vi "Controller Apply Soft Configuration.vi"(8 "error in (no error)":errorcluster, 11 "FOFB Configuration":T1={"FOFB Parameters"={"Network"={"FOFB Controller IP"="", "LNLS Control Network IP"="", "LNLS Control Network Power Supplies TCP Port"=0, "LNLS Control Network FOFB Configuration TCP Port"=0, "LNLS Control Network BPMs TCP Port"=0, "Monitoring Data TCP Port"=0, "Fast Archiver TCP Port"=0, "Fast Command TCP Port"=0, "TCP Listening Timeout"=0}, "Fast Acquisition"={"Sampling Period"=0, "Data Buffer Size"=0, "Monitoring Period"=0}, "Acquisition Network"=[], "Actuation Network"=[]}, "Number of Acquisition Chassis"=0, "Number of Actuation Chassis"=0, "Number of BPM Readings"=0, "BPM Reading Names"=[], "Selected BPM Readings"=[0, 1, 2, 3, 4, 5, 6, 7, 8, 9, 10, 11, 12, 13, 14, 15, 16, 17, 18, 19, 20, 21, 22, 23, 24, 25, 26, 27, 28, 29, 30, 31, 32, 33, 34, 35, 36, 37, 38, 39, 40, 41, 42, 43, 44, 45, 46, 47, 48, 49], "Number of Correctors"=0, "Corrector Names"=[], "Selected Correctors"=[0, 1, 2, 3, 4, 5, 6, 7, 8, 9, 10, 11, 12, 13, 14, 15, 16, 17, 18, 19, 20, 21, 22, 23, 24, 25, 26, 27, 28, 29, 30, 31, 32, 33, 34, 35, 36, 37, 38, 39, 40, 41, 42, 43, 44, 45, 46, 47, 48, 49], "Response Matrix"=[], "Reference Orbit"=[], "Correction Matrix"=[], "FPGA Filter Sets"=[], "Acquisition Chassis Names"=[], "Actuation Chassis Names"=[], "Acquisition Variables"=[], "Actuation Variables"=[], "PS Matrix Mapping"=[], "Inverse PS Matrix Mapping"=[], "BPM Matrix Mapping"=[], "Inverse BPM Matrix Mapping"=[], "BPM Planes"=[], "Corrector Planes"=[]}) -> (0 "error out":errorcluster, 3 "FOFB Configuration":T1={"FOFB Parameters"={"Network"={"FOFB Controller IP"="", "LNLS Control Network IP"="", "LNLS Control Network Power Supplies TCP Port"=0, "LNLS Control Network FOFB Configuration TCP Port"=0, "LNLS Control Network BPMs TCP Port"=0, "Monitoring Data TCP Port"=0, "Fast Archiver TCP Port"=0, "Fast Command TCP Port"=0, "TCP Listening Timeout"=0}, "Fast Acquisition"={"Sampling Period"=0, "Data Buffer Size"=0, "Monitoring Period"=0}, "Acquisition Network"=[], "Actuation Network"=[]}, "Number of Acquisition Chassis"=0, "Number of Actuation Chassis"=0, "Number of BPM Readings"=0, "BPM Reading Names"=[], "Selected BPM Readings"=[0, 1, 2, 3, 4, 5, 6, 7, 8, 9, 10, 11, 12, 13, 14, 15, 16, 17, 18, 19, 20, 21, 22, 23, 24, 25, 26, 27, 28, 29, 30, 31, 32, 33, 34, 35, 36, 37, 38, 39, 40, 41, 42, 43, 44, 45, 46, 47, 48, 49], "Number of Correctors"=0, "Corrector Names"=[], "Selected Correctors"=[0, 1, 2, 3, 4, 5, 6, 7, 8, 9, 10, 11, 12, 13, 14, 15, 16, 17, 18, 19, 20, 21, 22, 23, 24, 25, 26, 27, 28, 29, 30, 31, 32, 33, 34, 35, 36, 37, 38, 39, 40, 41, 42, 43, 44, 45, 46, 47, 48, 49], "Response Matrix"=[], "Reference Orbit"=[], "Correction Matrix"=[], "FPGA Filter Sets"=[], "Acquisition Chassis Names"=[], "Actuation Chassis Names"=[], "Acquisition Variables"=[], "Actuation Variables"=[], "PS Matrix Mapping"=[], "Inverse PS Matrix Mapping"=[], "BPM Matrix Mapping"=[], "Inverse BPM Matrix Mapping"=[], "BPM Planes"=[], "Corrector Planes"=[]})   [LabVIEW 2011, in "Controller VIs.lvlib"]
doc: "Performs tasks related with the FOFB configuration which does not require interrupting controller execution (ex.: load response matrix and reference orbit from file, calculate correction matrix, etc)."
uses:
  Controller VIs.lvlib
  Types Definitions/Type FOFB Configuration.ctl
  Types Definitions/Type FOFB Parameters.ctl
  Types Definitions/Type Network Configuration.ctl
  Types Definitions/Type FA Configuration.ctl
  Types Definitions/Type Acquisition Network Configuration.ctl
  Types Definitions/Type Actuation Network Configuration.ctl
  <vilib>/Utility/file.llb/Read From Spreadsheet File (DBL).vi
  File VIs.lvlib
  XML VIs.lvlib
  Type Definitions.lvlib
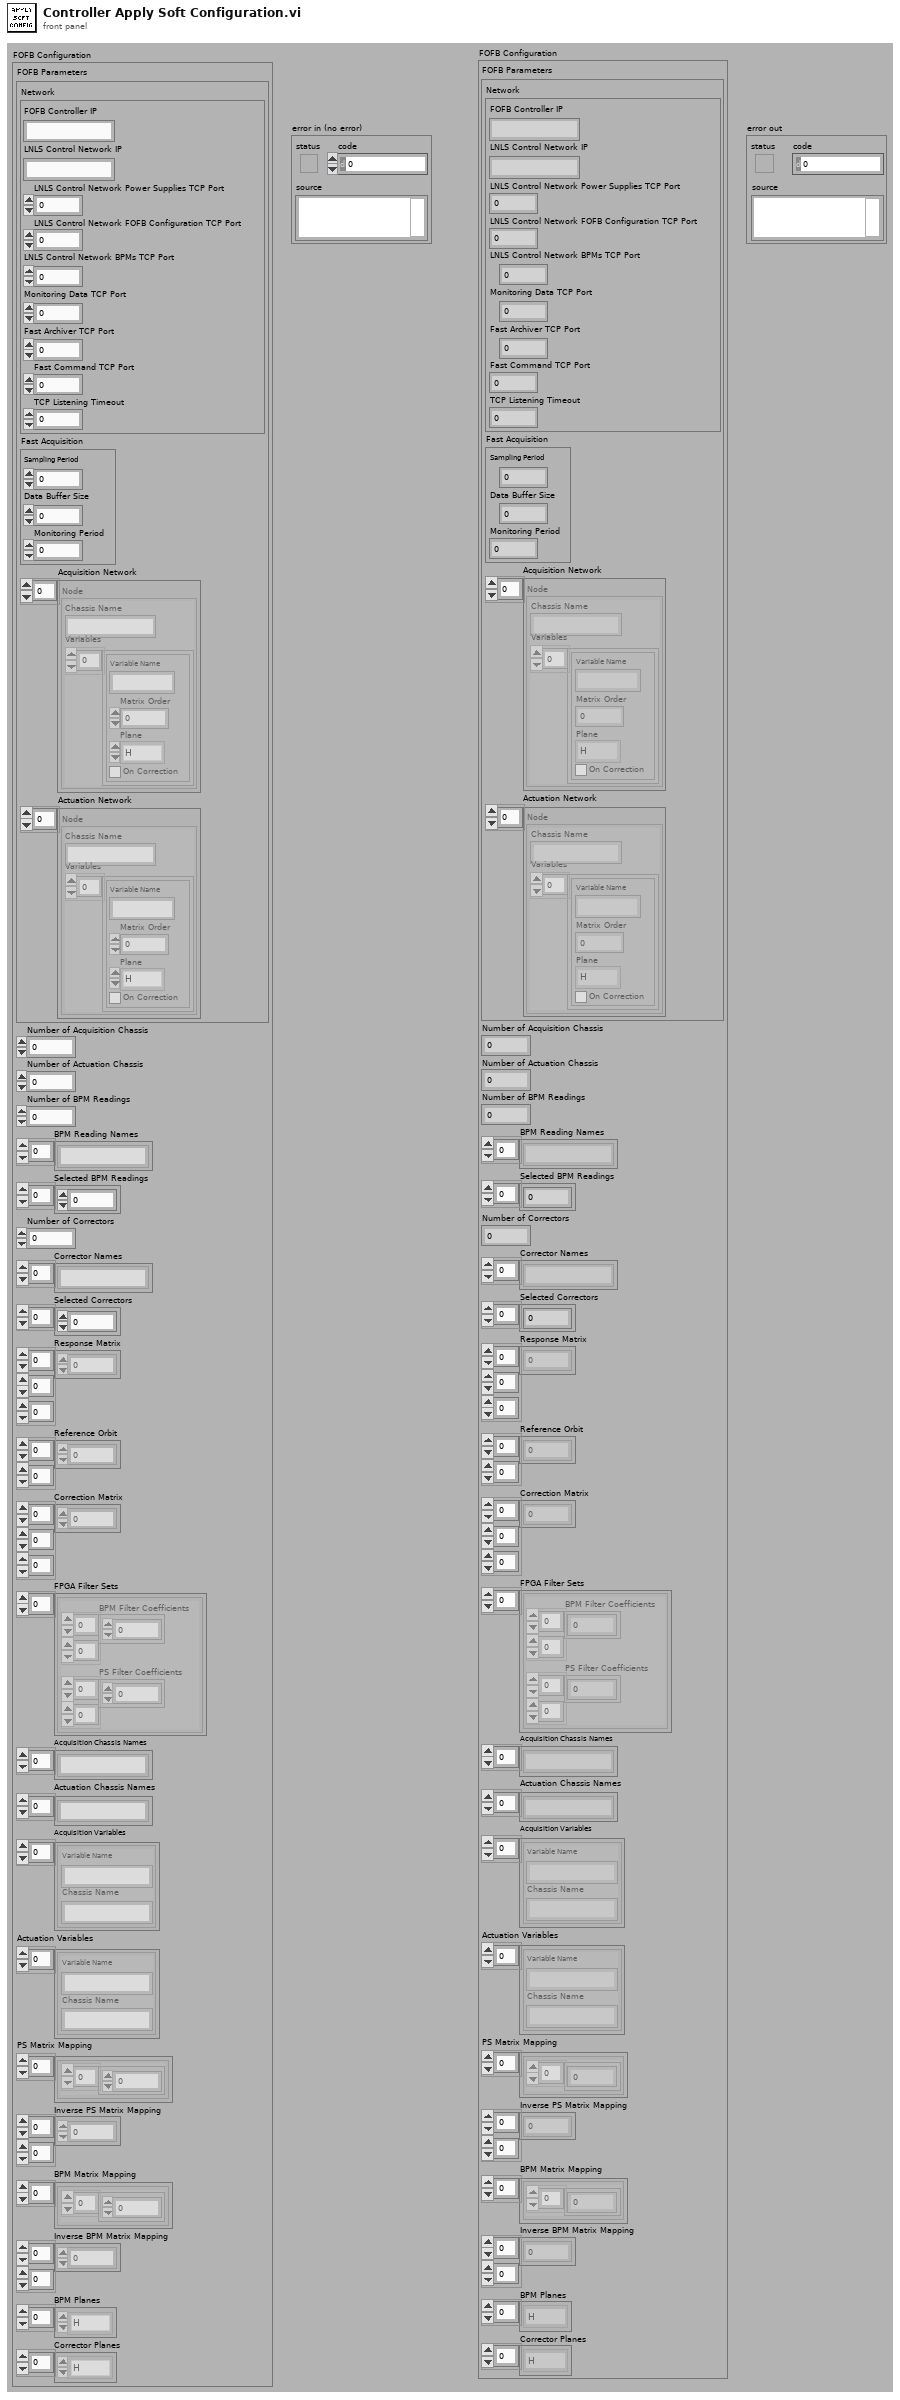
[diagram p1: front panel]
types:
  T1 = typedef "Type Definitions.lvlib/Type FOFB Configuration.ctl" = cluster{"FOFB Parameters":T2, "Number of Acquisition Chassis":i32, "Number of Actuation Chassis":i32, "Number of BPM Readings":i32, "BPM Reading Names":string[], "Selected BPM Readings":u32[], "Number of Correctors":i32, "Corrector Names":string[], "Selected Correctors":u32[], "Response Matrix":dbl[][][], "Reference Orbit":dbl[][], "Correction Matrix":dbl[][][], "FPGA Filter Sets":cluster{"BPM Filter Coefficients":dbl[][], "PS Filter Coefficients":dbl[][]}[], "Acquisition Chassis Names":string[], "Actuation Chassis Names":string[], "Acquisition Variables":cluster{"Variable Name":string, "Chassis Name":string}[], "Actuation Variables":cluster{"Variable Name":string, "Chassis Name":string}[], "PS Matrix Mapping":cluster{u32[]}[], "Inverse PS Matrix Mapping":u32[][], "BPM Matrix Mapping":cluster{u32[]}[], "Inverse BPM Matrix Mapping":u32[][], "BPM Planes":enum8{"H", "V"}[], "Corrector Planes":enum8{"H", "V"}[]}
  T2 = typedef "Type Definitions.lvlib/Type FOFB Parameters.ctl" = cluster{"Network":T3, "Fast Acquisition":T4, "Acquisition Network":T5, "Actuation Network":T6}
  T3 = typedef "Type Definitions.lvlib/Type Network Configuration.ctl" = cluster{"FOFB Controller IP":string, "LNLS Control Network IP":string, "LNLS Control Network Power Supplies TCP Port":u16, "LNLS Control Network FOFB Configuration TCP Port":u16, "LNLS Control Network BPMs TCP Port":u16, "Monitoring Data TCP Port":u16, "Fast Archiver TCP Port":u16, "Fast Command TCP Port":u16, "TCP Listening Timeout":i32}
  T4 = typedef "Type Definitions.lvlib/Type FA Configuration.ctl" = cluster{"Sampling Period":u32, "Data Buffer Size":u32, "Monitoring Period":u32}
  T5 = typedef "Type Definitions.lvlib/Type Acquisition Network Configuration.ctl" = cluster{"Chassis Name":string, "Variables":cluster{"Variable Name":string, "Matrix Order":u32, "Plane":enum8{"H", "V"}, "On Correction":bool}[]}[]
  T6 = typedef "Type Definitions.lvlib/Type Actuation Network Configuration.ctl" = cluster{"Chassis Name":string, "Variables":cluster{"Variable Name":string, "Matrix Order":u32, "Plane":enum8{"H", "V"}, "On Correction":bool}[]}[]
  T7 = typedef "Type Definitions.lvlib/Type BPM Parameters.ctl" = cluster{"Plane":enum8{"H", "V"}, "On Correction":bool}
  T8 = typedef "Type Definitions.lvlib/Type PS Parameters.ctl" = cluster{"Plane":enum8{"H", "V"}, "On Correction":bool}
  T9 = cluster{"BPM Filter Coefficients":dbl[][], "PS Filter Coefficients":dbl[][]}
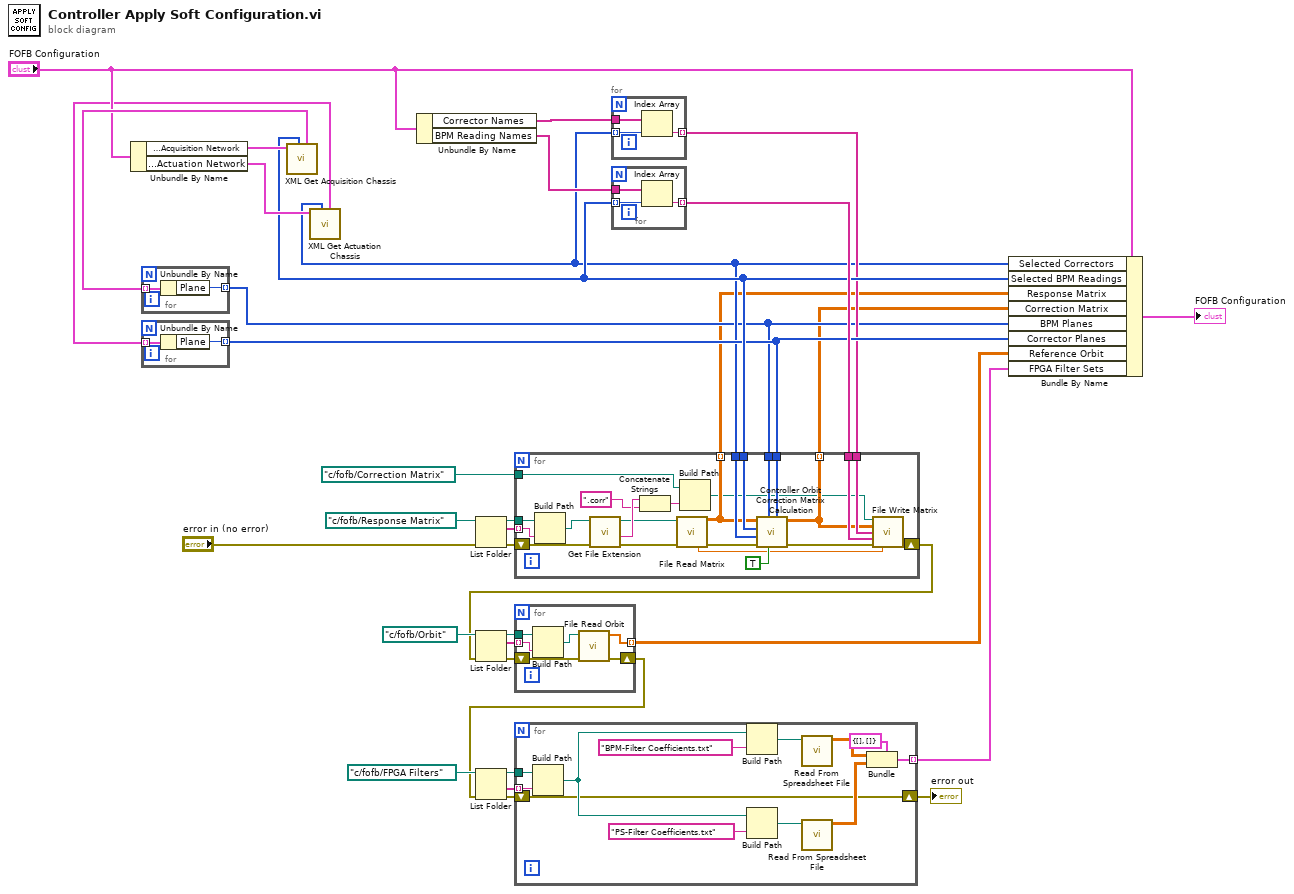
[diagram p0: block diagram]
diagram:
  n1 = Unbundle By Name("FOFB Configuration") -> ("FOFB Parameters.Acquisition Network"=w33:T5, "FOFB Parameters.Actuation Network"=w34:T6)
  n2 = call "XML Get Acquisition Chassis.vi"("Acquisition Network"=w33) -> ("BPM Parameters"=w35:T7[], "Selected BPM Readings"=w16:u32[])  [unwired: 4 in, 5 out]
  n3 = for {
    tunnel: w35 -> [w37] mode=indexing
    tunnel: [w36] -> w11 mode=indexing
    n4 = Unbundle By Name(w37) -> ("Plane"=w36:enum8{"H", "V"})
  }
  n5 = call "XML Get Actuation Chassis.vi"("Actuation Network"=w34) -> ("PS Parameters"=w18:T8[], "Selected Correctors"=w12:u32[])  [unwired: 4 in, 5 out]
  n6 = for {
    tunnel: w18 -> [w39] mode=indexing
    tunnel: [w38] -> w15 mode=indexing
    n7 = Unbundle By Name(w39) -> ("Plane"=w38:enum8{"H", "V"})
  }
  n8 = Unbundle By Name("FOFB Configuration") -> ("Corrector Names"=w14:string[], "BPM Reading Names"=w30:string[])
  n9 = List Folder(path=path "c:/fofb/Response Matrix", error in="error in (no error)") -> (path out=w19:path, filenames=w21:string[], error out=w9:errorcluster)  [unwired: 2 in, 1 out]
  n10 = for {
    tunnel: w12 -> [w41] mode=indexing
    tunnel: w14 -> [w42]
    tunnel: [w40] -> w13 mode=indexing
    n11 = Index Array(array=w42, index=w41) -> (element=w40:string)
  }
  n12 = for {
    tunnel: w16 -> [w44] mode=indexing
    tunnel: w30 -> [w45]
    tunnel: [w43] -> w17 mode=indexing
    n13 = Index Array(array=w45, index=w44) -> (element=w43:string)
  }
  n14 = for {
    tunnel: w19 -> [w49]
    tunnel: w21 -> [w69] mode=indexing
    tunnel: w15 -> [w64]
    tunnel: w11 -> [w63]
    tunnel: w13 -> [w62]
    tunnel: w17 -> [w61]
    tunnel: w16 -> [w60]
    tunnel: w12 -> [w59]
    tunnel: [w57] -> w3 mode=indexing
    tunnel: [w56] -> w2 mode=indexing
    tunnel: path "c:/fofb/Correction Matrix" ("path") -> [w48]
    shift-right: [w58] -> w8
    shift-left: w9 -> [w51]
    n15 = Build Path(base path=w49, name or relative path=w69) -> (appended path=w55:path)
    n16 = call <vilib>:"Get File Extension.vi"("error in (no error)"=w51, "file"=w55) -> ("error out"=w50:errorcluster, "filename without extension"=w54:string, "dup file"=w46:path)  [unwired: 6 in, 1 out]
    n17 = Concatenate Strings(w54, ".corr" ("string")) -> (w52:string)
    n18 = call "File Read Matrix.vi"("file path (dialog if empty)"=w46, "error in (no error)"=w50) -> ("Matrix"=w56:dbl[][], "Beam Energy (MeV)"=w67:dbl, "error out"=w65:errorcluster)  [unwired: 9 in, 2 out]
    n19 = Build Path(base path=w48, name or relative path=w52) -> (appended path=w47:path)
    n20 = call "Controller Orbit Correction Matrix Calculation.vi"("Corrector Planes"=w64, "Decouple H-V? (true)"=TRUE, "BPM Reading Planes"=w63, "error in (no error)"=w65, "Selected Correctors"=w59, "Selected BPM Readings"=w60, "Response Matrix"=w56) -> ("error out"=w66:errorcluster, "Correction Matrix"=w57:dbl[][])  [unwired: 3 in]
    n21 = call "File Write Matrix.vi"("file path (dialog if empty)"=w47, "Matrix"=w57, "Row Names"=w62, "Column Names"=w61, "error in (no error)"=w66, "Beam Energy (MeV)"=w67) -> ("error out"=w58:errorcluster)  [unwired: 9 in]
  }
  n22 = List Folder(path=path "c:/fofb/Orbit", error in=w8) -> (path out=w25:path, filenames=w23:string[], error out=w7:errorcluster)  [unwired: 2 in, 1 out]
  n23 = for {
    tunnel: w25 -> [w75]
    tunnel: w23 -> [w74] mode=indexing
    tunnel: [w72] -> w22 mode=indexing
    shift-right: [w70] -> w6
    shift-left: w7 -> [w71]
    n24 = Build Path(base path=w75, name or relative path=w74) -> (appended path=w73:path)
    n25 = call "File Read Orbit.vi"("error in (no error)"=w71, "file path (dialog if empty)"=w73) -> ("error out"=w70:errorcluster, "Orbit"=w72:dbl[])  [unwired: 7 in, 1 out]
  }
  n26 = List Folder(path=path "c:/fofb/FPGA Filters", error in=w6) -> (path out=w27:path, folder names=w29:string[], error out=w5:errorcluster)  [unwired: 2 in, 1 out]
  n27 = for {
    tunnel: w29 -> [w78] mode=indexing
    tunnel: w27 -> [w82]
    tunnel: [w79] -> w26 mode=indexing
    shift-right: [w76] -> w4
    shift-left: w5 -> [w76]
    n28 = Build Path(base path=w82, name or relative path=w78) -> (appended path=w85:path)
    n29 = Build Path(base path=w85, name or relative path="BPM-Filter Coefficients.txt" ("format string")) -> (appended path=w84:path)
    n30 = Build Path(base path=w85, name or relative path="PS-Filter Coefficients.txt" ("format string")) -> (appended path=w83:path)
    n31 = call-poly <vilib>:"Read From Spreadsheet File.vi"("file path (dialog if empty)"=w84) -> ("all rows"=w81:dbl[][])  [unwired: 6 in, 4 out]
    n32 = call-poly <vilib>:"Read From Spreadsheet File.vi"("file path (dialog if empty)"=w83) -> ("all rows"=w80:dbl[][])  [unwired: 6 in, 4 out]
    n33 = Bundle(cluster=T9 {"BPM Filter Coefficients"=[], "PS Filter Coefficients"=[]}, "BPM Filter Coefficients"=w81, "PS Filter Coefficients"=w80) -> (w79:T9)
  }
  "error out" <- w4
  n34 = Bundle By Name(cluster="FOFB Configuration", "Selected Correctors"=w12, "Selected BPM Readings"=w16, "Response Matrix"=w2, "Correction Matrix"=w3, "BPM Planes"=w11, "Corrector Planes"=w15, "Reference Orbit"=w22, "FPGA Filter Sets"=w26) -> (→"FOFB Configuration":T1)
